vi "ex_setTdmProperty.vi"   [LabVIEW 2020]
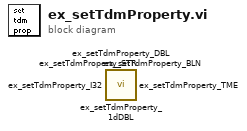
[diagram p0: block diagram]
diagram:
  n1 = call <vilib>:"ex_setTdmProperty_1dDBL.vi"() -> ()  [unwired: 7 in, 1 out]
  n2 = call <vilib>:"ex_setTdmProperty_BLN.vi"() -> ()  [unwired: 7 in, 1 out]
  n3 = call <vilib>:"ex_setTdmProperty_I32.vi"() -> ()  [unwired: 7 in, 1 out]
  n4 = call <vilib>:"ex_setTdmProperty_TME.vi"() -> ()  [unwired: 7 in, 1 out]
  n5 = call <vilib>:"ex_setTdmProperty_DBL.vi"() -> ()  [unwired: 7 in, 1 out]
  n6 = call <vilib>:"ex_setTdmProperty_STR.vi"() -> ()  [unwired: 7 in, 1 out]
